vi "DemoPathSearch.vi"() -> ()   [LabVIEW 2018]
panel:
  in  "Look-Ahead Time (s)":dbl=0.25
  out "Velocity Goal":dbl(slide) scale=-20.0..20.0
  out "Robot Position":cluster{dbl[], dbl[]}[](graph)
  out "closest point":i32
  out "iout":i32
  out "index look ahead pt":i32
  in  "robot x":dbl
  in  "robot y":dbl
  in  "is":i32
  out "Data (index by column)":dbl[][](array[numeric])
  # "distance, time, x, y velocity, orientation,"
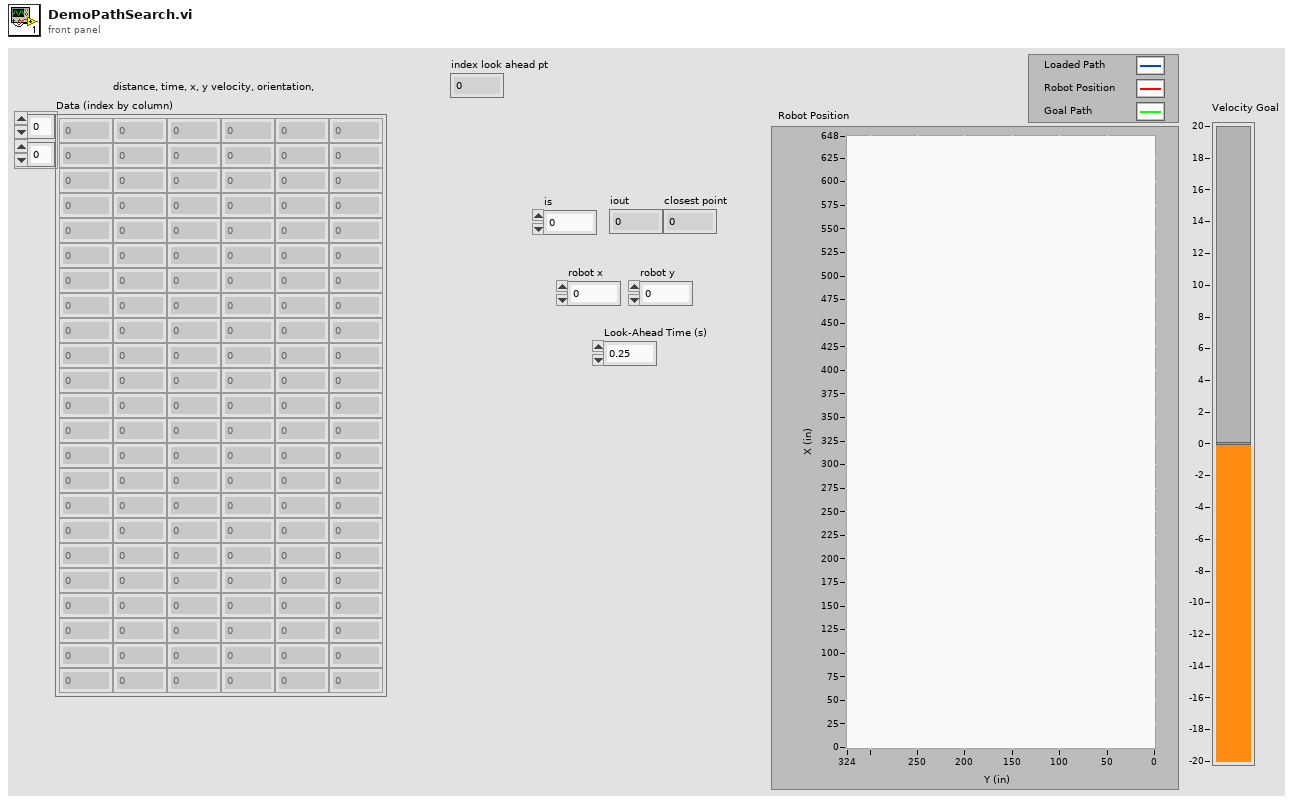
[diagram p1: front panel]
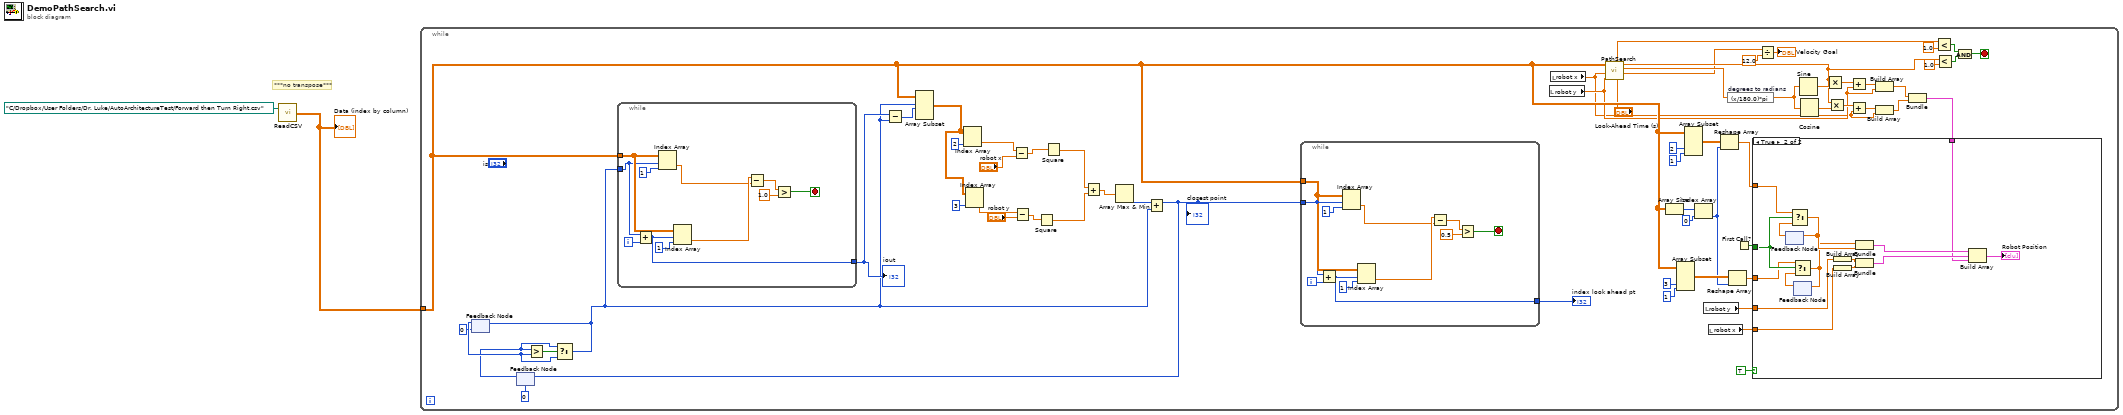
[diagram p0: block diagram]
diagram:
  # "***no transpose***"
  n1 = call "ReadCSV.vi"("File Path (.csv)"=path "C:/Dropbox/User Folders/Dr. Luke/AutoArchitectureTest/Forward then Turn Right.csv") -> ("Data (index by row)"=w1:dbl[][])  [unwired: 1 in]
  "Data (index by column)" <- w1
  n2 = while {
    tunnel: w1 -> [w32]
    stop <- w7 stop-if-true
    n3 = feedback #1(0) -> (w46:i32)
    n4 = feedback #2(0) -> (w45:i32)
    n5 = Greater?(x=w45, y=w46) -> (0:w47:bool)
    n6 = Select(t=w45, s=w47, f=w46) -> (s? t:f=w43:i32)
    n7 = feedback-in #1(w43) -> ()
    n8 = while {
      tunnel: w32 -> [w101]
      tunnel: [w92] -> w50
      tunnel: w43 -> [w93]
      i -> [w95]
      stop <- w94 stop-if-true
      n9 = Add(x=w93, y=w95) -> (x+y=w92:i32)
      n10 = Index Array(array=w101, index (row)=w93, index (col)=1 ("index")) -> (element=w96:dbl)
      n11 = Index Array(array=w101, index (row)=w92, index (col)=1 ("index")) -> (element=w97:dbl)
      n12 = Subtract(x=w97, y=w96) -> (x-y=w99:dbl)
      n13 = Greater?(x=w99, y=1.0) -> (0:w94:bool)
    }
    "iout" <- w50
    n14 = Subtract(x=w50, y=w43) -> (x-y=w49:i32)
    n15 = Array Subset(array=w32, index (row)=w43, length (row)=w49) -> (w52:dbl[][])  [unwired: 2 in]
    n16 = Index Array(array=w52, index (col)=2 ("disabled index (col)")) -> (element=w62:dbl[])  [unwired: 1 in]
    n17 = Index Array(array=w52, index (col)=3 ("disabled index (col)")) -> (element=w59:dbl[])  [unwired: 1 in]
    n18 = Subtract(x=w62, y="robot x") -> (x-y=w58:dbl[])
    n19 = Subtract(x=w59, y="robot y") -> (x-y=w57:dbl[])
    n20 = Square(x=w57) -> (x^2=w55:dbl[])
    n21 = Square(x=w58) -> (x^2=w56:dbl[])
    n22 = Add(x=w56, y=w55) -> (x+y=w54:dbl[])
    n23 = Array Max & Min(array=w54) -> (min index (indices)=w64:i32)  [unwired: 3 out]
    n24 = Add(x=w64, y=w43) -> (x+y=w51:i32)
    "closest point" <- w51
    n25 = feedback-in #2(w51) -> ()
    n26 = while {
      tunnel: [w82] -> _
      tunnel: [w81] -> w48
      tunnel: w32 -> [w83]
      tunnel: w51 -> [w82]
      i -> [w84]
      stop <- w87 stop-if-true
      n27 = Add(x=w82, y=w84) -> (x+y=w81:i32)
      n28 = Index Array(array=w83, index (row)=w82, index (col)=1 ("index")) -> (element=w85:dbl)
      n29 = Index Array(array=w83, index (row)=w81, index (col)=1 ("index")) -> (element=w86:dbl)
      n30 = Subtract(x=w86, y=w85) -> (x-y=w89:dbl)
      n31 = Greater?(x=w89, y=0.5) -> (0:w87:bool)
    }
    "index look ahead pt" <- w48
    n32 = local read "robot y"() -> (w19:dbl)
    n33 = local read "robot x"() -> (w17:dbl)
    n34 = call "PathSearch.vi"("Look-Ahead Time (s)"="Look-Ahead Time (s)", "Robot Y (in)"=w19, "Robot X (in)"=w17, "Path"=w32) -> ("Velocity Goal (in/s)"=w4:dbl, "Angle To Goal (deg)"=w26:dbl, "Distance to Goal (in)"=w8:dbl, "Distance from End (in)"=w13:dbl)  [unwired: 2 in, 2 out]
    n35 = Array Size(array=w32) -> (size(s)=w31:i32[])
    n36 = Array Subset(array=w32, index (col)=3 ("index"), length (col)=1 ("length")) -> (w33:dbl[][])  [unwired: 2 in]
    n37 = Array Subset(array=w32, index (col)=2 ("index"), length (col)=1 ("length")) -> (w36:dbl[][])  [unwired: 2 in]
    n38 = Index Array(array=w31, index=0) -> (element=w29:i32)
    n39 = local read "robot y"() -> (w28:dbl)
    n40 = local read "robot x"() -> (w27:dbl)
    n41 = Reshape Array(w36, w29) -> (w35:dbl[])
    n42 = expression code="(x/180.0)*pi" "degrees to radians"(w26) -> (w25:dbl)
    n43 = Reshape Array(w33, w29) -> (w34:dbl[])
    n44 = First Call?() -> (First Call?: T/F=w37:bool)
    n45 = Divide(x=w4, y=12.0) -> (x/y=→"Velocity Goal":dbl)
    n46 = Sine(x=w25) -> (sin(x)=w24:dbl)
    n47 = Cosine(x=w25) -> (cos(x)=w23:dbl)
    n48 = Multiply(x=w8, y=w24) -> (x*y=w22:dbl)
    n49 = Multiply(x=w8, y=w23) -> (x*y=w21:dbl)
    n50 = Add(x=w22, y=w19) -> (x+y=w20:dbl)
    n51 = Add(x=w21, y=w17) -> (x+y=w18:dbl)
    n52 = Build Array(w20, w19) -> (w16:dbl[])
    n53 = Build Array(w18, w17) -> (w15:dbl[])
    n54 = Bundle(w16, w15) -> (w14:cluster{dbl[], dbl[]})  [unwired: 1 in]
    n55 = case shown="True" TRUE {
      tunnel: w37 -> [_ w78]
      tunnel: w35 -> [_ w77]
      tunnel: w34 -> [_ w75]
      tunnel: w28 -> [_ w68]
      tunnel: w27 -> [_ w67]
      tunnel: w14 -> [_ w66]
      frame False {
      }
      frame True {
        n56 = feedback #3() -> (w79:dbl[])  [unwired: 1 in]
        n57 = Select(t=w77, s=w78, f=w79) -> (s? t:f=w76:dbl[])
        n58 = feedback-in #3(w76) -> ()
        n59 = feedback #4() -> (w80:dbl[])  [unwired: 1 in]
        n60 = Select(t=w75, s=w78, f=w80) -> (s? t:f=w74:dbl[])
        n61 = feedback-in #4(w74) -> ()
        n62 = Build Array(w68) -> (w70:dbl[])
        n63 = Build Array(w67) -> (w69:dbl[])
        n64 = Bundle(w74, w76) -> (w73:cluster{dbl[], dbl[]})  [unwired: 1 in]
        n65 = Bundle(w70, w69) -> (w71:cluster{dbl[], dbl[]})  [unwired: 1 in]
        n66 = Build Array(w73, w71, w66) -> (→"Robot Position":cluster{dbl[], dbl[]}[])
      }
    }
    n67 = Less?(x=w13, y=1.0) -> (x < y?=w11:bool)
    n68 = Less?(x=w8, y=1.0) -> (x < y?=w9:bool)
    n69 = And(x=w11, y=w9) -> (x .and. y?=w7:bool)
  }
